vi "get bootloader version.vi"(7 "Release":u32, 8 "error in (no error)":errorcluster, 9 "Minor":u32, 10 "Major":u32, 11 "id":i32) -> (0 "error out":errorcluster, 1 "Minor out":u32, 2 "Major out":u32, 3 "function return":i32, 5 "Release out":u32)   [LabVIEW 2012, in "libximc.lvlib"]
doc: "result_t XIMC_API get_bootloader_version (device_t id, unsigned int* Major, unsigned int* Minor, unsigned int* Release);"
uses:
  libximc.lvlib
  libximc.dll
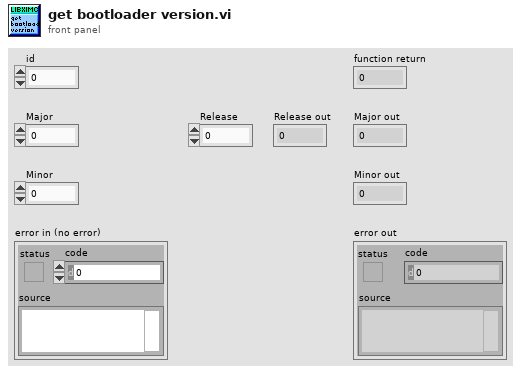
[diagram p1: front panel]
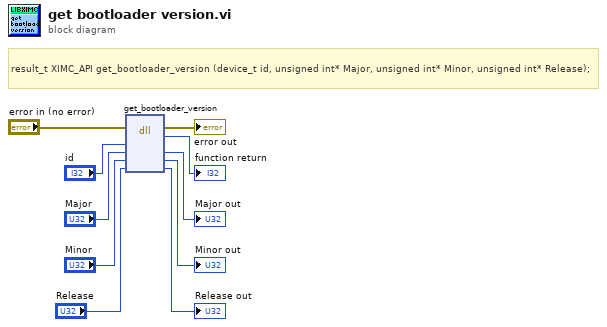
[diagram p0: block diagram]
diagram:
  # "result_t XIMC_API get_bootloader_version (device_t id, unsigned int* Major, unsigned int* Minor, unsigned int* Release);"
  n1 = dll-call lib="C:/Users/user/Desktop/labview-2.9.11-gen/libximc.*" fn="get_bootloader_version"(error in="error in (no error)", "id"="id", "Major"="Major", "Minor"="Minor", "Release"="Release") -> (error out=→"error out":errorcluster, →"function return":i32, "Major"=→"Major out":u32, "Minor"=→"Minor out":u32, "Release"=→"Release out":u32)  [unwired: 3 in, 1 out]
